vi "Onto.vi"(6 "Old":bool[](array[boolean]), 9 "Onto":bool[](array[boolean]), 11 "Refs cluster In":T1) -> (1 "Changed":bool, 3 "Refs cluster Out":T1, 4 "New":bool[](array[boolean]), 5 "Trigger array":bool[](array[boolean]))   [LabVIEW 2015]
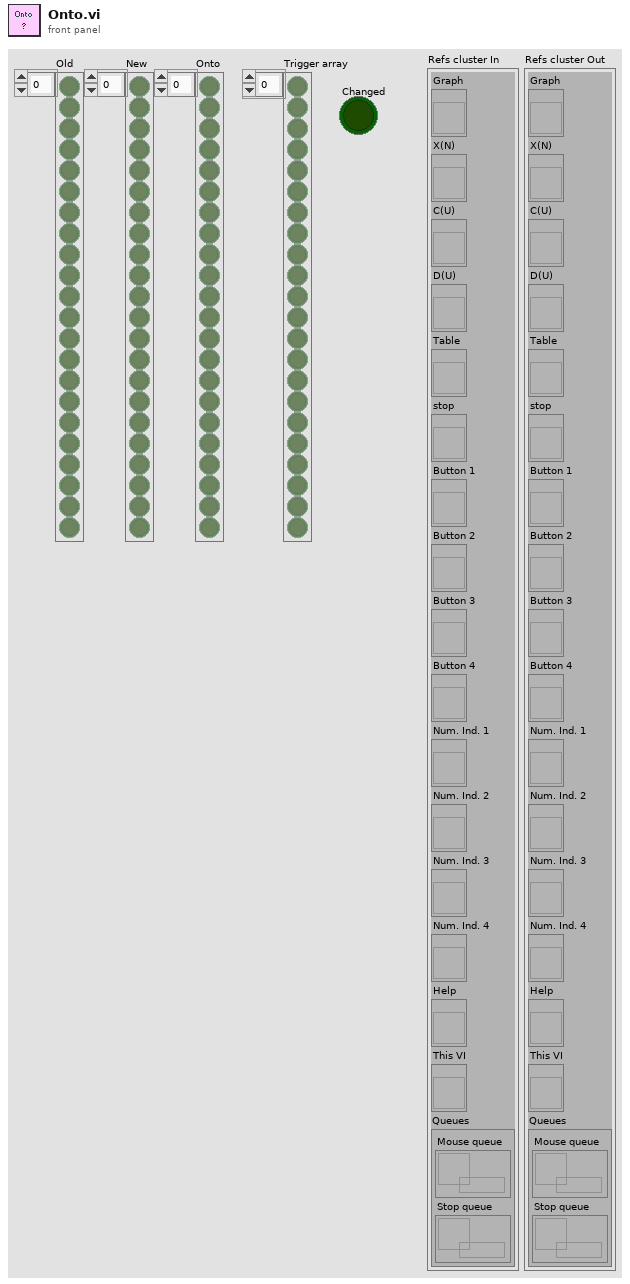
[diagram p1: front panel]
types:
  T1 = cluster{"Graph":refnum<vi>, "X(N)":refnum<vi>, "C(U)":refnum<vi>, "D(U)":refnum<vi>, "Table":refnum<vi>, "stop":refnum<vi>, "Button 1":refnum<vi>, "Button 2":refnum<vi>, "Button 3":refnum<vi>, "Button 4":refnum<vi>, "Num. Ind. 1":refnum<vi>, "Num. Ind. 2":refnum<vi>, "Num. Ind. 3":refnum<vi>, "Num. Ind. 4":refnum<vi>, "Help":refnum<vi>, "This VI":refnum<vi>, "Queues":cluster{"Mouse queue":refnum<queue>, "Stop queue":refnum<queue>}}
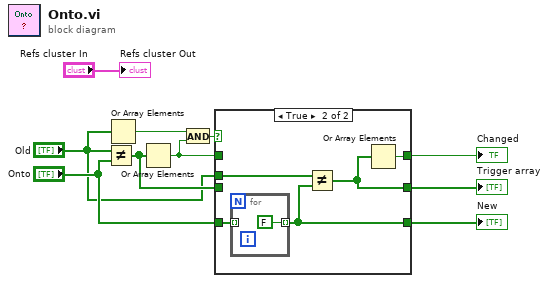
[diagram p0: block diagram]
diagram:
  n1 = Not Equal?(x="Old", y="Onto") -> (x != y?=w6:bool[])
  n2 = Or Array Elements(Boolean array="Old") -> (logical OR=w10:bool)
  n3 = Or Array Elements(Boolean array=w6) -> (logical OR=w8:bool)
  n4 = And(x=w10, y=w8) -> (x .and. y?=w9:bool)
  n5 = case shown="True" w9 {
    tunnel: "Onto" -> [w12 w18]
    tunnel: [w12 w14] -> w3
    tunnel: w8 -> [w13 _]
    tunnel: [w13 w15] -> w1
    tunnel: w6 -> [w11 _]
    tunnel: [w11 w16] -> w4
    tunnel: "Old" -> [_ w17]
    frame False {
    }
    frame True {
      n6 = for {
        tunnel: w18 -> [_] mode=indexing
        tunnel: [FALSE] -> w14 mode=indexing
      }
      n7 = Not Equal?(x=w17, y=w14) -> (x != y?=w16:bool[])
      n8 = Or Array Elements(Boolean array=w16) -> (logical OR=w15:bool)
    }
  }
  "Changed" <- w1
  "Trigger array" <- w4
  "New" <- w3
  "Refs cluster Out" <- "Refs cluster In"
